vi "PM100D_Get-Wave.vi"(0 "VISA in":refnum<visa-resource-name>, 11 "error in (no error)":errorcluster) -> (2 "WAV_MAX":dbl, 4 "VISA out":refnum<visa-resource-name>, 8 "WAV":dbl, 13 "WAV_MIN":dbl, 15 "error out":errorcluster)   [LabVIEW 2011]
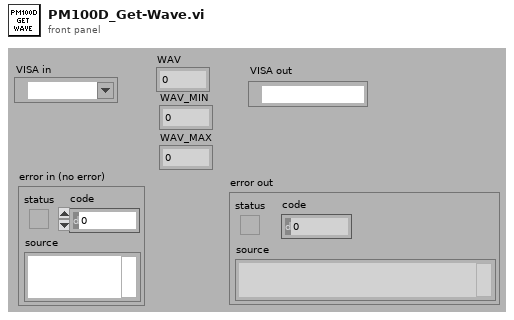
[diagram p1: front panel]
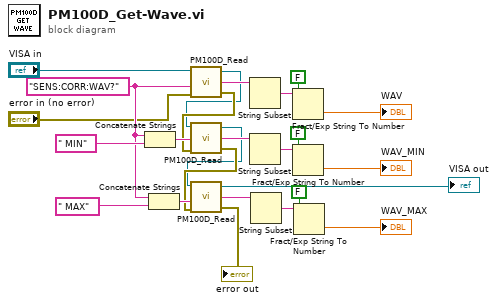
[diagram p0: block diagram]
diagram:
  w11 = "SENS:CORR:WAV?" ("Command")
  n1 = Concatenate Strings(w11, " MIN" ("string")) -> (w14:string)
  n2 = Concatenate Strings(w11, " MAX" ("string")) -> (w12:string)
  n3 = call "PM100D_Read.vi"("error in (no error)"="error in (no error)", "Command"=w11, "VISA in"="VISA in") -> ("error out"=w5:errorcluster, "ReadValue"=w22:string, "VISA out"=w2:refnum<visa-resource-name>)  [unwired: 1 in]
  n4 = call "PM100D_Read.vi"("error in (no error)"=w5, "Command"=w14, "VISA in"=w2) -> ("error out"=w4:errorcluster, "ReadValue"=w16:string, "VISA out"=w1:refnum<visa-resource-name>)  [unwired: 1 in]
  n5 = call "PM100D_Read.vi"("error in (no error)"=w4, "Command"=w12, "VISA in"=w1) -> ("error out"=→"error out":errorcluster, "ReadValue"=w15:string, "VISA out"=→"VISA out":refnum<visa-resource-name>)  [unwired: 1 in]
  n6 = String Subset(string=w22) -> (substring=w23:string)  [unwired: 2 in]
  n7 = String Subset(string=w16) -> (substring=w19:string)  [unwired: 2 in]
  n8 = String Subset(string=w15) -> (substring=w17:string)  [unwired: 2 in]
  n9 = Fract/Exp String To Number(use system decimal point (T)=FALSE, string=w23) -> (number=→"WAV":dbl)  [unwired: 2 in, 1 out]
  n10 = Fract/Exp String To Number(use system decimal point (T)=FALSE, string=w19) -> (number=→"WAV_MIN":dbl)  [unwired: 2 in, 1 out]
  n11 = Fract/Exp String To Number(use system decimal point (T)=FALSE, string=w17) -> (number=→"WAV_MAX":dbl)  [unwired: 2 in, 1 out]
